vi "TestDeadband.vi"() -> ()   [LabVIEW 2020]
panel:
  in  "stop":bool
  out "Output":dbl
  in  "Limit":dbl=0.1
  in  "Input":dbl
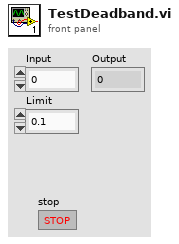
[diagram p1: front panel]
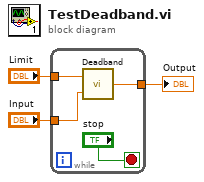
[diagram p0: block diagram]
diagram:
  n1 = while {
    tunnel: "Limit" -> [w7]
    tunnel: "Input" -> [w6]
    tunnel: [w5] -> w1
    stop <- "stop" stop-if-true
    n2 = call "Deadband.vi"("Limit"=w6, "Input"=w7) -> ("Output"=w5:dbl)
  }
  "Output" <- w1
